vi "HAL_Open.vi"(7 "Instrument Name":string, 8 "error in":errorcluster, 10 "Reset?":bool=TRUE, 11 "Alias":string) -> (0 "error out":errorcluster, 3 "Handle":T1)   [LabVIEW 2015]
uses:
  Handle.ctl
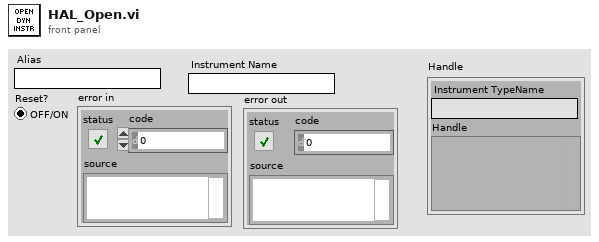
[diagram p1: front panel]
types:
  T1 = typedef "Handle.ctl" = cluster{"Instrument TypeName":string, "Handle":variant}
  T2 = cluster{"Instrument Name":string, "Handle":variant}
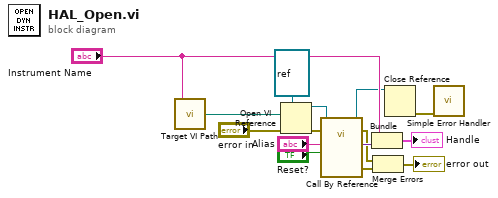
[diagram p0: block diagram]
diagram:
  n1 = call "Target VI Path.vi"("Instrument Name"="Instrument Name") -> ("Path to VI"=w1:path)
  n2 = Open VI Reference(type specifier VI Refnum (for type only)=refnum<vi> refnum, vi path=w1, error in (no error)="error in") -> (vi reference=w14:refnum<vi>, error out=w4:errorcluster)  [unwired: 3 in]
  n3 = call-by-ref "?"(reference=w14, error in=w4, "Reset?"="Reset?", "Alias"="Alias") -> (reference out=w8:refnum<vi>, error out=w5:errorcluster, 0:"error out"=w6:errorcluster, "Handle"=w11:variant)  [unwired: 8 in]
  n4 = Bundle("Instrument Name"="Instrument Name", "Handle"=w11) -> (→"Handle":T2)  [unwired: 1 in]
  n5 = Merge Errors(w5, w6) -> (→"error out":errorcluster)
  n6 = Close Reference(reference=w8) -> (error out=w7:errorcluster)  [unwired: 1 in]
  n7 = call <vilib>:"Simple Error Handler.vi"("error in (no error)"=w7) -> ()  [unwired: 4 in, 5 out]
